vi "SimpleParser.vi"(1 "Command":string) -> (0 "Response":string)   [LabVIEW 2015]
uses:
  SCLN_RW_Select.ctl
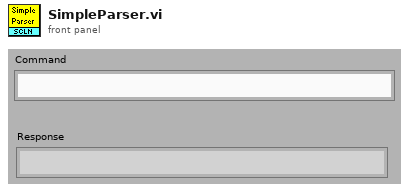
[diagram p1: front panel]
types:
  T1 = typedef "SCLN_RW_Select.ctl" = enum16{"Read", "Write"}
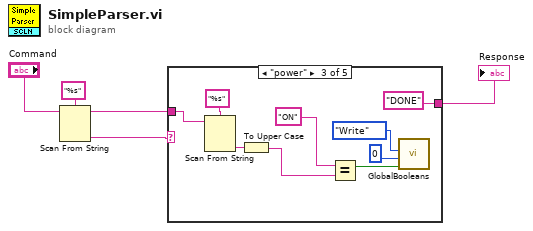
[diagram p0: block diagram]
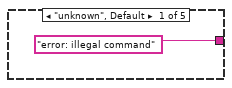
[diagram p2: hidden frame]
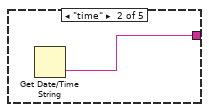
[diagram p3: hidden frame]
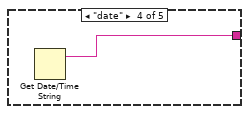
[diagram p4: hidden frame]
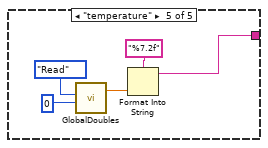
[diagram p5: hidden frame]
diagram:
  n1 = Scan From String(format string="%s" ("Format String"), input string="Command") -> (remaining string=w2:string, output 1=w1:string)  [unwired: 3 in, 2 out]
  n2 = case shown="\"power\"" w1 {
    tunnel: ["error: illegal command" ("time string") w7 "DONE" w17 w18] -> w5
    tunnel: w2 -> [_ _ w12 _ _]
    frame "unknown", Default {
    }
    frame "time" {
      n3 = Get Date/Time String() -> (time string=w7:string)  [unwired: 3 in, 1 out]
    }
    frame "power" {
      n4 = Scan From String(format string="%s" ("Format String"), input string=w12) -> (output 1=w11:string)  [unwired: 3 in, 3 out]
      n5 = To Upper Case(1:w11) -> (0:w9:string)
      n6 = Equal?(x="ON", y=w9) -> (x = y?=w8:bool)
      n7 = call "GlobalBooleans.vi"("Write Value"=w8, "Element"=0, "Operation"=SCLN_RW_Select."Write" ("GBL_RW")) -> ()  [unwired: 1 in, 2 out]
    }
    frame "date" {
      n8 = Get Date/Time String() -> (date string=w17:string)  [unwired: 3 in, 1 out]
    }
    frame "temperature" {
      n9 = call "GlobalDoubles.vi"("Element"=0, "Operation"=SCLN_RW_Select."Read" ("GBL_RW")) -> ("Read Value"=w19:dbl)  [unwired: 2 in, 1 out]
      n10 = Format Into String(format string="%7.2f", w19) -> (resulting string=w18:string)  [unwired: 2 in, 1 out]
    }
  }
  "Response" <- w5
